vi "BiasRej.vi"(4 "Bias Reject Mode":bool, 6 "BiasRejectON?":bool, 8 "Error In (No Error)":errorcluster, 9 "Fixed Voltage Rejection":string="VR0", 10 "Fixed Current Rejection":string="IR0", 11 "Potentiostat":refnum<visa-resource-name>="Solartron1287") -> (0 "Error Out":errorcluster, 3 "VISA Name Out":refnum<visa-resource-name>)   [LabVIEW 2018]
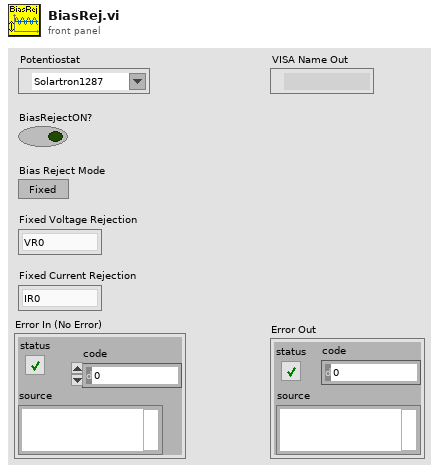
[diagram p1: front panel]
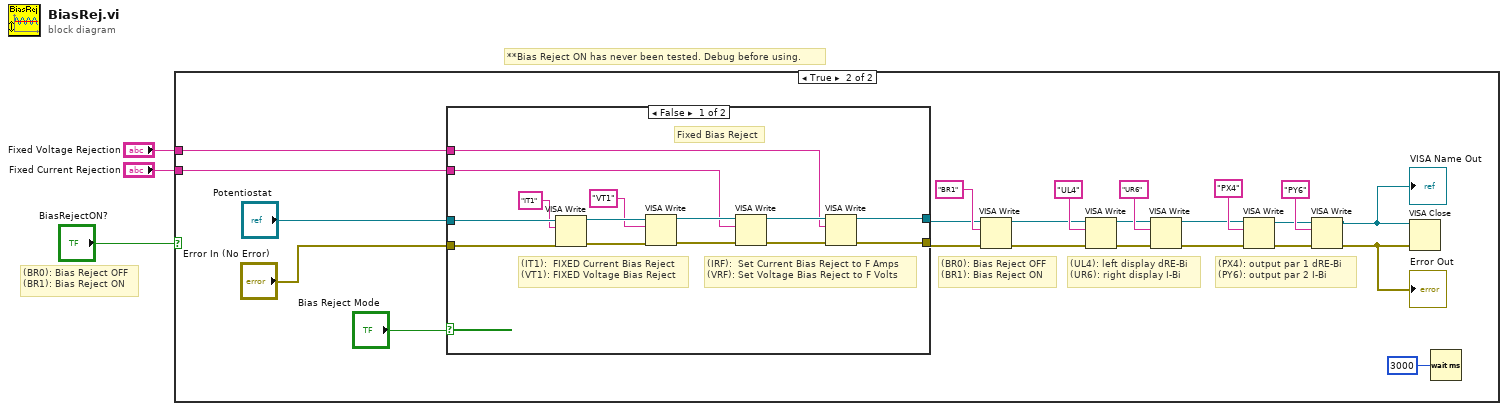
[diagram p0: block diagram]
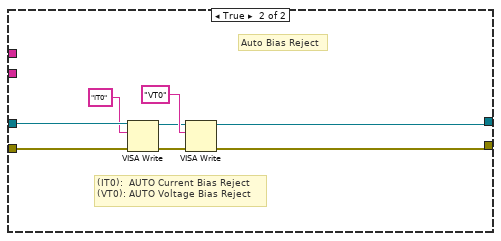
[diagram p3: hidden frame]
diagram:
  # "**Bias Reject ON has never been tested. Debug before using."
  # "(BR0): Bias Reject OFF\n(BR1): Bias Reject ON"
  n1 = case shown="True" "BiasRejectON?" {
    tunnel: "Fixed Current Rejection" -> [_ w25]
    tunnel: "Fixed Voltage Rejection" -> [_ w24]
    frame False {
      # "Do nothing:\nBR OFF (BR0) is the default setting applied in the Initialization VI"
    }
    frame True {
      # "(PX4): output par 1 dRE-Bi\n(PY6): output par 2 I-Bi"
      # "(UL4): left display dRE-Bi\n(UR6): right display I-Bi"
      # "(BR0): Bias Reject OFF\n(BR1): Bias Reject ON"
      n2 = case shown="False" "Bias Reject Mode" {
        tunnel: "Potentiostat" -> [w39 w48]
        tunnel: "Error In (No Error)" -> [w40 w47]
        tunnel: w25 -> [w30 _]
        tunnel: w24 -> [w29 _]
        tunnel: [w28 w42] -> w22
        tunnel: [w27 w41] -> w21
        frame False {
          # "(IRF):  Set Current Bias Reject to F Amps\n(VRF): Set Voltage Bias Reject to F Volts"
          # "(IT1):  FIXED Current Bias Reject\n(VT1): FIXED Voltage Bias Reject"
          # "Fixed Bias Reject"
          n3 = VISA Write(VISA resource name=w39, write buffer="IT1" ("y"), error in (no error)=w40) -> (VISA resource name out=w37:refnum<visa-resource-name>, error out=w38:errorcluster)  [unwired: 1 out]
          n4 = VISA Write(VISA resource name=w37, write buffer="VT1" ("y"), error in (no error)=w38) -> (VISA resource name out=w36:refnum<visa-resource-name>, error out=w35:errorcluster)  [unwired: 1 out]
          n5 = VISA Write(VISA resource name=w36, write buffer=w30, error in (no error)=w35) -> (VISA resource name out=w34:refnum<visa-resource-name>, error out=w33:errorcluster)  [unwired: 1 out]
          n6 = VISA Write(VISA resource name=w34, write buffer=w29, error in (no error)=w33) -> (VISA resource name out=w28:refnum<visa-resource-name>, error out=w27:errorcluster)  [unwired: 1 out]
        }
        frame True {
          # "(IT0):  AUTO Current Bias Reject\n(VT0): AUTO Voltage Bias Reject"
          # "Auto Bias Reject"
          n7 = VISA Write(VISA resource name=w48, write buffer="IT0" ("data"), error in (no error)=w47) -> (VISA resource name out=w44:refnum<visa-resource-name>, error out=w43:errorcluster)  [unwired: 1 out]
          n8 = VISA Write(VISA resource name=w44, write buffer="VT0" ("data"), error in (no error)=w43) -> (VISA resource name out=w42:refnum<visa-resource-name>, error out=w41:errorcluster)  [unwired: 1 out]
        }
      }
      n9 = VISA Write(VISA resource name=w22, write buffer="BR1" ("y"), error in (no error)=w21) -> (VISA resource name out=w16:refnum<visa-resource-name>, error out=w15:errorcluster)  [unwired: 1 out]
      n10 = VISA Write(VISA resource name=w16, write buffer="UL4" ("y"), error in (no error)=w15) -> (VISA resource name out=w13:refnum<visa-resource-name>, error out=w12:errorcluster)  [unwired: 1 out]
      n11 = VISA Write(VISA resource name=w13, write buffer="UR6" ("y"), error in (no error)=w12) -> (VISA resource name out=w10:refnum<visa-resource-name>, error out=w9:errorcluster)  [unwired: 1 out]
      n12 = VISA Write(VISA resource name=w10, write buffer="PX4" ("y"), error in (no error)=w9) -> (VISA resource name out=w7:refnum<visa-resource-name>, error out=w6:errorcluster)  [unwired: 1 out]
      n13 = VISA Write(VISA resource name=w7, write buffer="PY6" ("y"), error in (no error)=w6) -> (VISA resource name out=w5:refnum<visa-resource-name>, error out=w4:errorcluster)  [unwired: 1 out]
      "Error Out" <- w4
      "VISA Name Out" <- w5
      n14 = VISA Close(VISA resource name=w5, error in (no error)=w4) -> ()  [unwired: 1 out]
      n15 = Wait (ms)(milliseconds to wait=u32 3000) -> ()  [unwired: 1 out]
    }
  }
